vi "calculate.vi"(11 "Input":T1) -> (3 "Output":T1)   [LabVIEW 2022 SP3]
uses:
  SM_Data.ctl
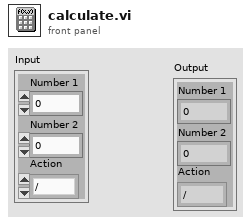
[diagram p1: front panel]
types:
  T1 = typedef "SM_Data.ctl" = cluster{"Number 1":dbl, "Number 2":dbl, "Action":enum16{"/", "*", "-", "+", " "}}
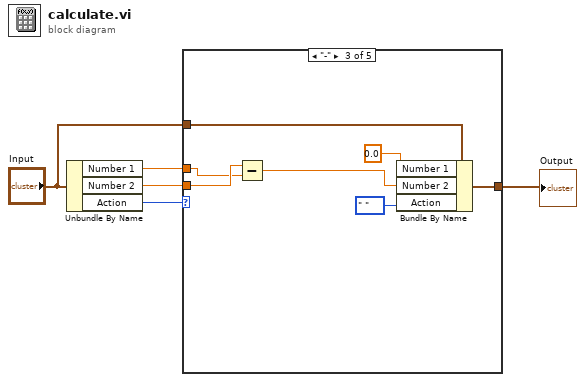
[diagram p0: block diagram]
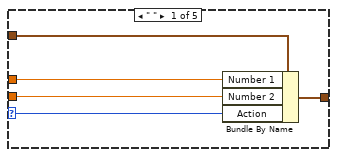
[diagram p2: hidden frame]
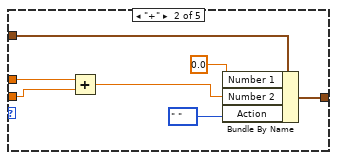
[diagram p3: hidden frame]
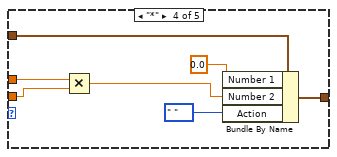
[diagram p4: hidden frame]
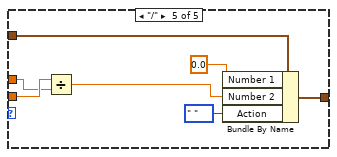
[diagram p5: hidden frame]
diagram:
  n1 = Unbundle By Name("Input") -> ("Number 1"=w3:dbl, "Number 2"=w4:dbl, "Action"=w5:enum16{"/", "*", "-", "+", " "})
  n2 = case shown="\"-\"" w5 {
    selector: w5 -> [w7 _ _ _ _]
    tunnel: w4 -> [w8 w14 w21 w27 w35]
    tunnel: w3 -> [w9 w15 w20 w28 w34]
    tunnel: "Input" -> [w10 w17 w24 w31 w38]
    tunnel: [w6 w16 w23 w30 w37] -> w1
    frame " " {
      n3 = Bundle By Name(cluster=w10, "Number 1"=w9, "Number 2"=w8, "Action"=w7) -> (w6:T1)
    }
    frame "+" {
      n4 = Add(x=w15, y=w14) -> (x+y=w13:dbl)
      n5 = Bundle By Name(cluster=w17, "Number 1"=0.0, "Number 2"=w13, "Action"=enum16{"/", "*", "-", "+", " "}." ") -> (w16:T1)
    }
    frame "-" {
      n6 = Subtract(x=w21, y=w20) -> (x-y=w19:dbl)
      n7 = Bundle By Name(cluster=w24, "Number 1"=0.0, "Number 2"=w19, "Action"=enum16{"/", "*", "-", "+", " "}." ") -> (w23:T1)
    }
    frame "*" {
      n8 = Multiply(x=w28, y=w27) -> (x*y=w26:dbl)
      n9 = Bundle By Name(cluster=w31, "Number 1"=0.0, "Number 2"=w26, "Action"=enum16{"/", "*", "-", "+", " "}." ") -> (w30:T1)
    }
    frame "/" {
      n10 = Divide(x=w35, y=w34) -> (x/y=w33:dbl)
      n11 = Bundle By Name(cluster=w38, "Number 1"=0.0, "Number 2"=w33, "Action"=enum16{"/", "*", "-", "+", " "}." ") -> (w37:T1)
    }
  }
  "Output" <- w1
